vi "appendCircNumArr.vi"(7 "Buffer Length":i32, 8 "error in (no error)":errorcluster, 9 "New Numeric":dbl, 10 "Numeric Array":dbl[](array[numeric]), 11 "MatOper in":refnum<class "MatOper.lvclass">) -> (0 "error out":errorcluster, 2 "Updated Numeric Array":dbl[](array[numeric]), 3 "MatOper out":refnum<class "MatOper.lvclass">)   [LabVIEW 2016, in "OfcFunc.lvlib" / "MatOper.lvclass"]
doc: "Append the circular numeric array based on the buffer length."
uses:
  MatOper.lvclass
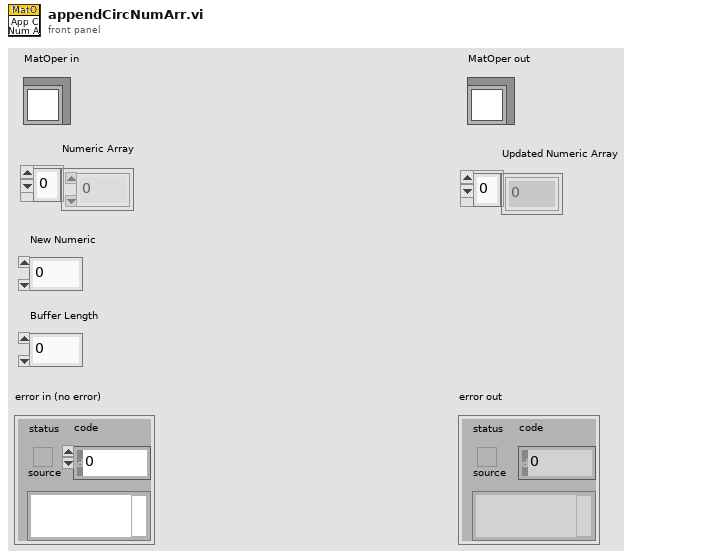
[diagram p1: front panel]
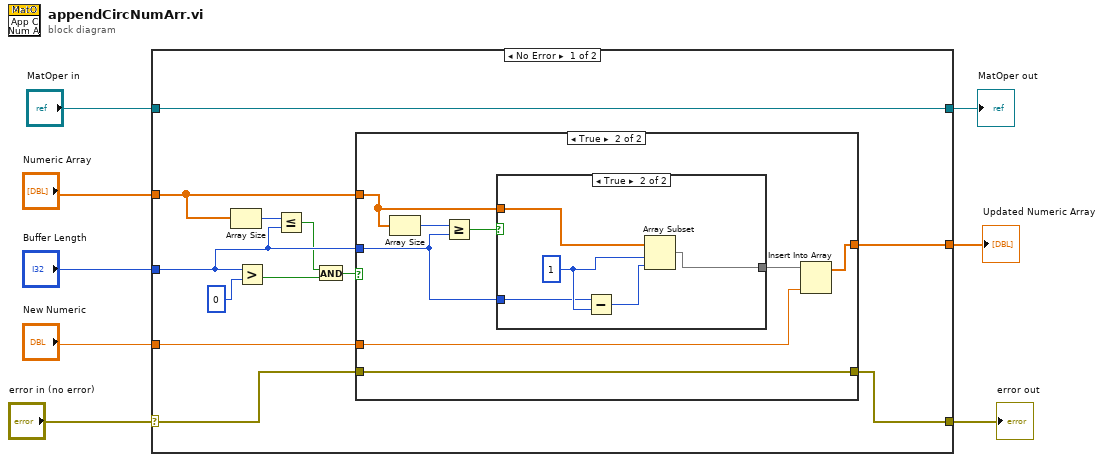
[diagram p0: block diagram]
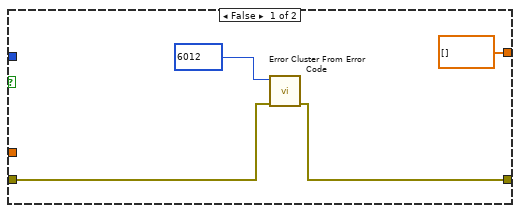
[diagram p2: hidden frame]
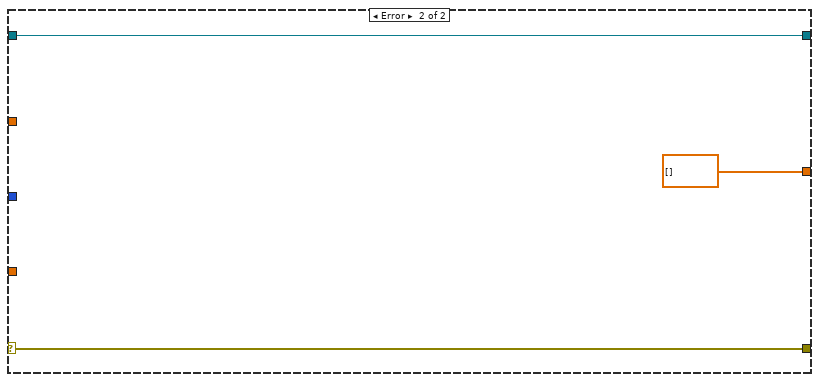
[diagram p4: hidden frame]
diagram:
  n1 = case shown="No Error" "error in (no error)" {
    selector: "error in (no error)" -> [w16 w41]
    tunnel: [w15 w41] -> w7
    tunnel: [w20 w40] -> w5
    tunnel: "MatOper in" -> [w20 w40]
    tunnel: "Numeric Array" -> [w14 _]
    tunnel: "Buffer Length" -> [w12 _]
    tunnel: "New Numeric" -> [w18 _]
    tunnel: [w17 dbl[] [] ("Numeric Array")] -> w1
    frame No Error {
      n2 = Array Size(array=w14) -> (size(s)=w13:i32)
      n3 = Greater?(x=w12, y=0) -> (0:w9:bool)
      n4 = Less Or Equal?(x=w13, y=w12) -> (x <= y?=w10:bool)
      n5 = And(x=w10, y=w9) -> (x .and. y?=w11:bool)
      n6 = case shown="True" w11 {
        tunnel: w14 -> [_ w30]
        tunnel: w18 -> [_ w26]
        tunnel: [dbl[] [] ("Numeric Array") w28] -> w17
        tunnel: w12 -> [_ w27]
        tunnel: w16 -> [w23 w25]
        tunnel: [w22 w25] -> w15
        frame False {
          n7 = call <vilib>:"Error Cluster From Error Code.vi"("error in (no error)"=w23, "error code (0)"=6012) -> ("error out"=w22:errorcluster)  [unwired: 7 in]
        }
        frame True {
          n8 = Array Size(array=w30) -> (size(s)=w32:i32)
          n9 = Greater Or Equal?(x=w32, y=w27) -> (x >= y?=w31:bool)
          n10 = case shown="True" w31 {
            tunnel: w30 -> [w33 w38]
            tunnel: [w33 w34] -> w29
            tunnel: w27 -> [_ w36]
            frame False {
            }
            frame True {
              w37 = 1 ("index")
              n11 = Subtract(x=w36, y=w37) -> (x-y=w35:i32)
              n12 = Array Subset(array=w38, index=w37, length=w35) -> (w34:dbl[])
            }
          }
          n13 = Insert Into Array(array=w29, new element=w26) -> (w28:dbl[])  [unwired: 1 in]
        }
      }
    }
    frame Error {
    }
  }
  "error out" <- w7
  "MatOper out" <- w5
  "Updated Numeric Array" <- w1
